vi "myRIO v1.0 Build MUX Configuration DI Block.vi"(11 "DI (N Samples) Channel List":T4) -> (3 "Channel Reservation List":T1)   [LabVIEW 2021]
uses:
  <vilib>/myRIO/Common/Instrument Driver Framework/myRIO v1.0/DI Block/typedefs/DI Block Channels List.ctl
  <vilib>/myRIO/Common/Instrument Driver Framework/myRIO v1.0/DI Block/typedefs/DI Block Channels Enum.ctl
  <vilib>/myRIO/Common/Instrument Driver Framework/myRIO v1.0/Resource Manager/typedefs/myRIO v1.0 Channel Reservation List.ctl
  <vilib>/myRIO/Common/Instrument Driver Framework/myRIO v1.0/Resource Manager/typedefs/myRIO v1.0 Channel Reservation Info.ctl
  <vilib>/myRIO/Common/Instrument Driver Framework/myRIO v1.0/Resource Manager/typedefs/myRIO v1.0 Connector List.ctl
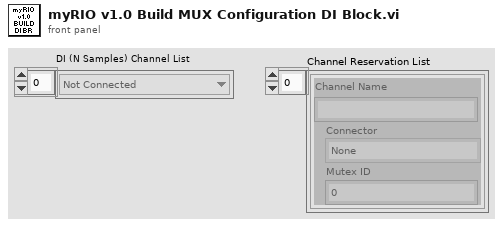
[diagram p1: front panel]
types:
  T1 = typedef "myRIO v1.0 Channel Reservation List.ctl" = T2[]
  T2 = typedef "myRIO v1.0 Channel Reservation Info.ctl" = cluster{"Channel Name":string, "Connector":T3, "Mutex ID":i32}
  T3 = typedef "myRIO v1.0 Connector List.ctl" = enum32{"None", "ConnectorA", "ConnectorB", "ConnectorC"}
  T4 = typedef "DI Block Channels List.ctl" = T5[]
  T5 = typedef "DI Block Channels Enum.ctl" = enum16{"Not Connected", "A/DI0 (N Samples)", "A/DI1 (N Samples)", "A/DI2 (N Samples)", "A/DI3 (N Samples)", "A/DI4 (N Samples)", "A/DI5 (N Samples)", "A/DI6 (N Samples)", "A/DI7 (N Samples)", "A/DI8 (N Samples)", "A/DI9 (N Samples)", "A/DI10 (N Samples)", "A/DI11 (N Samples)", "A/DI12 (N Samples)", "A/DI13 (N Samples)", "A/DI14 (N Samples)", "A/DI15 (N Samples)", "A/DI16 (N Samples)", "A/DI17 (N Samples)", "A/DI18 (N Samples)", "A/DI19 (N Samples)", "B/DI0 (N Samples)", "B/DI1 (N Samples)", "B/DI2 (N Samples)", "B/DI3 (N Samples)", "B/DI4 (N Samples)", "B/DI5 (N Samples)", "B/DI6 (N Samples)", "B/DI7 (N Samples)", "B/DI8 (N Samples)", "B/DI9 (N Samples)", "B/DI10 (N Samples)", "B/DI11 (N Samples)", "B/DI12 (N Samples)", "B/DI13 (N Samples)", "B/DI14 (N Samples)", "B/DI15 (N Samples)", "B/DI16 (N Samples)", "B/DI17 (N Samples)", "B/DI18 (N Samples)", "B/DI19 (N Samples)"}
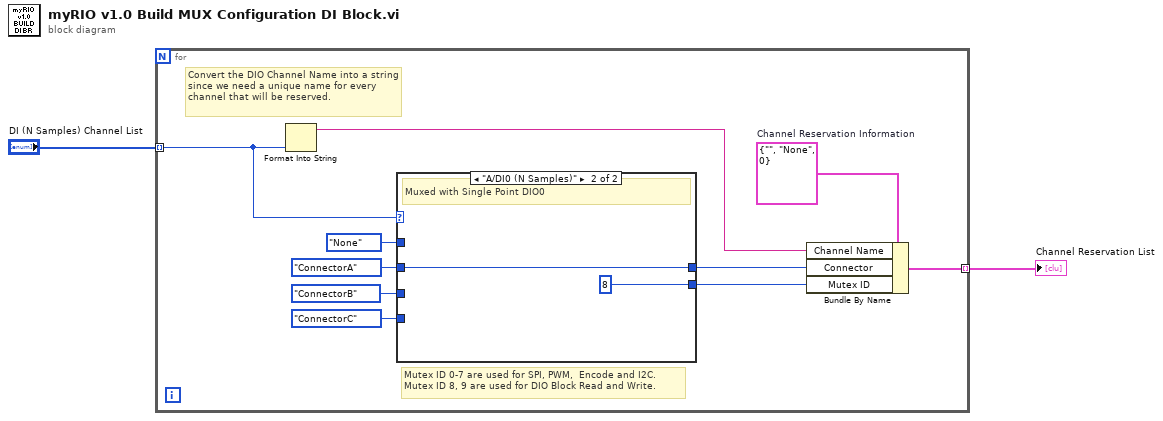
[diagram p0: block diagram]
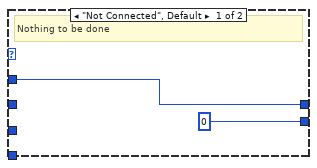
[diagram p2: hidden frame]
diagram:
  n1 = for {
    tunnel: "DI (N Samples) Channel List" -> [w6] mode=indexing
    tunnel: [w7] -> w1 mode=indexing
    w10 = T2 {"Channel Name"="", "Connector"=enum."None", "Mutex ID"=0}  # Channel Reservation Information
    # "Mutex ID 0-7 are used for SPI, PWM,  Encode and I2C.\nMutex ID 8, 9 are used for DIO Block Read and Write."
    # "Convert the DIO Channel Name into a string since we need a unique name for every channel that will be reserved."
    n2 = Format Into String(w6) -> (resulting string=w5:string)  [unwired: 3 in, 1 out]
    n3 = case shown="\"A/DI0 (N Samples)\"" w6 {
      tunnel: myRIO_v1.0_Connector_List."None" ("Connector List") -> [w14 _]
      tunnel: myRIO_v1.0_Connector_List."ConnectorA" ("Connector List") -> [_ w15]
      tunnel: [0 ("index") 8 ("index")] -> w8
      tunnel: [w14 w15] -> w9
      tunnel: myRIO_v1.0_Connector_List."ConnectorB" ("Connector List") -> [_ _]
      tunnel: myRIO_v1.0_Connector_List."ConnectorC" ("Connector List") -> [_ _]
      frame "Not Connected", Default {
        # "Nothing to be done"
      }
      frame "A/DI0 (N Samples)" {
        # "Muxed with Single Point DIO0"
      }
    }
    n4 = Bundle By Name(cluster=w10, "Channel Name"=w5, "Connector"=w9, "Mutex ID"=w8) -> (w7:T2)
  }
  "Channel Reservation List" <- w1
